vi "SRV_Update Replies Indicator.vi"(0 "Replies ref":refnum<vi>, 7 "Text to Append":string, 11 "error in (no error)":errorcluster) -> (4 "Replies ref out":refnum<vi>, 15 "error out":errorcluster)   [LabVIEW 2009]
doc: "Updates the string indicator referenced by \"Replies ref\". Autoscrolls to the show the last lines when an update is made.\n\n\nAuthor: Mike Schultz - Logic PD"
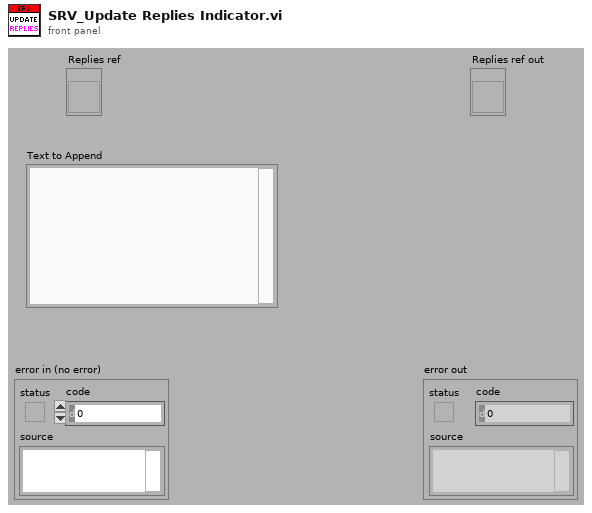
[diagram p1: front panel]
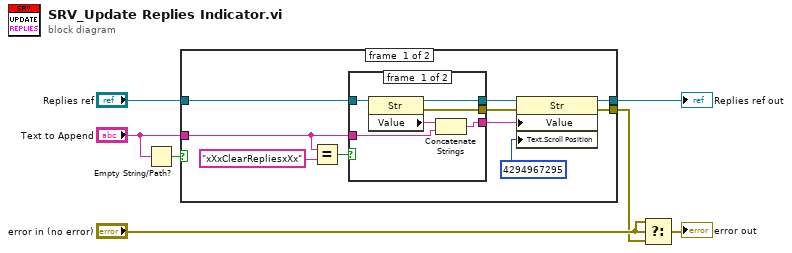
[diagram p0: block diagram]
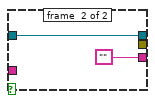
[diagram p2: hidden frame]
diagram:
  n1 = Empty String/Path?(string/path="Text to Append") -> (empty?=w5:bool)
  n2 = case shown="False" w5 {
    tunnel: "Replies ref" -> [w12 w26]
    tunnel: [w17 w26] -> w6
    tunnel: [w16 _] -> w1
    tunnel: "Text to Append" -> [w8 _]
    frame #0 {
      n3 = Equal?(x=w8, y="xXxClearRepliesxXx") -> (x = y?=w14:bool)
      n4 = case shown="False" w14 {
        tunnel: [w23 _] -> w13
        tunnel: w12 -> [w21 w25]
        tunnel: [w22 w25] -> w11
        tunnel: [w20 ""] -> w10
        tunnel: w8 -> [w19 _]
        frame #0 {
          n5 = property class="Str"(reference=w21) -> (reference out=w22:refnum<vi>, error out=w23:errorcluster, "Value"=w18:string)  [unwired: 1 in]
          n6 = Concatenate Strings(w18, w19) -> (w20:string)
        }
        frame #1 {
        }
      }
      n7 = property class="Str"(reference=w11, error in=w13, "Value"=w10, "Text.Scroll Position"=u32 4294967295) -> (reference out=w17:refnum<vi>, error out=w16:errorcluster)
    }
    frame #1 {
    }
  }
  "Replies ref out" <- w6
  n8 = Select(t="error in (no error)", s="error in (no error)", f=w1) -> (s? t:f=→"error out":errorcluster)
